vi "classes.vi"(0 "HGF_FGV_Factory":refnum<class "HGF_FGV_Factory.lvclass">, 1 "className":string, 5 "error in (no error)":errorcluster) -> (14 "dup HGF_FGV_Factory":refnum<class "HGF_FGV_Factory.lvclass">, 16 "Object":refnum<class>, 19 "error out":errorcluster)   [LabVIEW 2012, in "HGF_FGV.lvlib" / "HGF_FGV_Factory.lvclass"]
doc: "This dynamaic dispatch VI contains constant objects of all classes that can be produced by HGF_Factory.\nClass has to be defined by name. \n\nOptionally, you can also specifiy a Class Path String instead, but you have to make sure that all dependencies are available.\n\nChild classes have to override it to define additional classes."
uses:
  HGF_FGV_Factory.lvclass
  HGF_FGV_Append/HGF_FGV_Append.lvclass
  HGF_FGV_Clear/HGF_FGV_Clear.lvclass
  HGF_FGV_Delete/HGF_FGV_Delete.lvclass
  HGF_FGV_Index/HGF_FGV_Index.lvclass
  HGF_FGV_Insert/HGF_FGV_Insert.lvclass
  HGF_FGV_Replace/HGF_FGV_Replace.lvclass
  HGF_FGV_SelectByName/HGF_FGV_SelectByName.lvclass
  HGF_FGV_Selection/HGF_FGV_Selection.lvclass
  HGF_FGV_Size/HGF_FGV_Size.lvclass
  HGF_FGV_Subset/HGF_FGV_SubSet.lvclass
  HGF_FGV_VisitAll/HGF_FGV_VisitAll.lvclass
  HGF_FGV_VisitByName/HGF_FGV_VisitByName.lvclass
  HGF_FGV_VisitSelection/HGF_FGV_VisitSelection.lvclass
  HGF_FGV_VisitSubset/HGF_FGV_VisitSubSet.lvclass
  HGF_Factory/HGF_Factory.lvclass
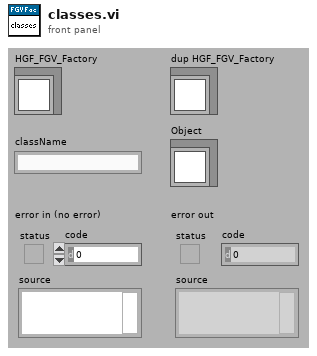
[diagram p1: front panel]
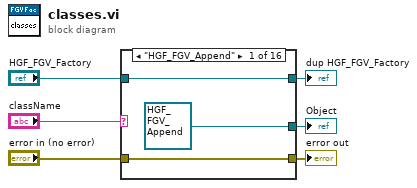
[diagram p0: block diagram]
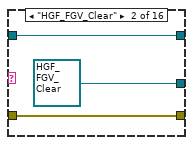
[diagram p2: hidden frame]
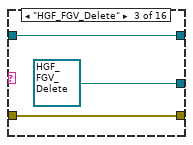
[diagram p3: hidden frame]
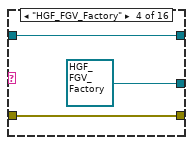
[diagram p4: hidden frame]
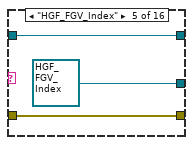
[diagram p5: hidden frame]
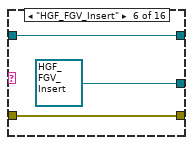
[diagram p6: hidden frame]
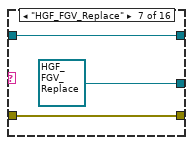
[diagram p7: hidden frame]
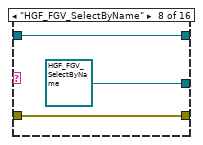
[diagram p8: hidden frame]
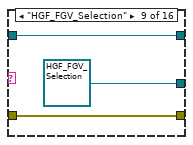
[diagram p9: hidden frame]
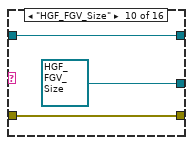
[diagram p10: hidden frame]
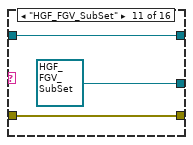
[diagram p11: hidden frame]
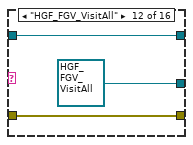
[diagram p12: hidden frame]
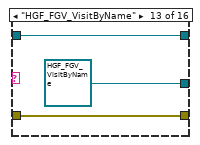
[diagram p13: hidden frame]
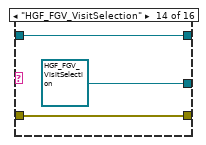
[diagram p14: hidden frame]
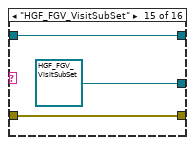
[diagram p15: hidden frame]
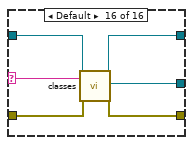
[diagram p16: hidden frame]
diagram:
  n1 = case shown="\"HGF_FGV_Append\"" "className" {
    selector: "className" -> [_ _ _ _ _ _ _ _ _ _ _ _ _ _ _ w54]
    tunnel: [refnum<class "HGF_FGV_Append.lvclass"> refnum ("HGF_FGV.lvlib:HGF_FGV_Append.lvclass") refnum<class "HGF_FGV_Clear.lvclass"> refnum ("HGF_FGV.lvlib:HGF_FGV_Clear.lvclass") refnum<class "HGF_FGV_Delete.lvclass"> refnum ("HGF_FGV.lvlib:HGF_FGV_Delete.lvclass") refnum<class "HGF_FGV_Factory.lvclass"> refnum ("HGF_FGV.lvlib:HGF_FGV_Factory.lvclass") refnum<class "HGF_FGV_Index.lvclass"> refnum ("HGF_FGV.lvlib:HGF_FGV_Index.lvclass") refnum<class "HGF_FGV_Insert.lvclass"> refnum ("HGF_FGV.lvlib:HGF_FGV_Insert.lvclass") refnum<class "HGF_FGV_Replace.lvclass"> refnum ("HGF_FGV.lvlib:HGF_FGV_Replace.lvclass") refnum<class "HGF_FGV_SelectByName.lvclass"> refnum ("HGF_FGV.lvlib:HGF_FGV_SelectByName.lvclass") refnum<class "HGF_FGV_Selection.lvclass"> refnum ("HGF_FGV.lvlib:HGF_FGV_Selection.lvclass") refnum<class "HGF_FGV_Size.lvclass"> refnum ("HGF_FGV.lvlib:HGF_FGV_Size.lvclass") refnum<class "HGF_FGV_SubSet.lvclass"> refnum ("HGF_FGV.lvlib:HGF_FGV_SubSet.lvclass") refnum<class "HGF_FGV_VisitAll.lvclass"> refnum ("HGF_FGV.lvlib:HGF_FGV_VisitAll.lvclass") refnum<class "HGF_FGV_VisitByName.lvclass"> refnum ("HGF_FGV.lvlib:HGF_FGV_VisitByName.lvclass") refnum<class "HGF_FGV_VisitSelection.lvclass"> refnum ("HGF_FGV.lvlib:HGF_FGV_VisitSelection.lvclass") refnum<class "HGF_FGV_VisitSubSet.lvclass"> refnum ("HGF_FGV.lvlib:HGF_FGV_VisitSubSet.lvclass") w55] -> w3
    tunnel: "error in (no error)" -> [w7 w10 w13 w17 w19 w22 w25 w28 w31 w34 w37 w40 w43 w46 w49 w57]
    tunnel: [w7 w10 w13 w17 w19 w22 w25 w28 w31 w34 w37 w40 w43 w46 w49 w56] -> w5
    tunnel: "HGF_FGV_Factory" -> [w8 w11 w14 w18 w20 w23 w26 w29 w32 w35 w38 w41 w44 w47 w50 w53]
    tunnel: [w8 w11 w14 w18 w20 w23 w26 w29 w32 w35 w38 w41 w44 w47 w50 w52] -> w1
    frame "HGF_FGV_Append" {
    }
    frame "HGF_FGV_Clear" {
    }
    frame "HGF_FGV_Delete" {
    }
    frame "HGF_FGV_Factory" {
    }
    frame "HGF_FGV_Index" {
    }
    frame "HGF_FGV_Insert" {
    }
    frame "HGF_FGV_Replace" {
    }
    frame "HGF_FGV_SelectByName" {
    }
    frame "HGF_FGV_Selection" {
    }
    frame "HGF_FGV_Size" {
    }
    frame "HGF_FGV_SubSet" {
    }
    frame "HGF_FGV_VisitAll" {
    }
    frame "HGF_FGV_VisitByName" {
    }
    frame "HGF_FGV_VisitSelection" {
    }
    frame "HGF_FGV_VisitSubSet" {
    }
    frame Default {
      n2 = call-parent "classes.vi"("HGF_Factory"=w53, "className"=w54, "error in (no error)"=w57) -> ("HGF_Factory dup"=w52:refnum<class "HGF_FGV_Factory.lvclass">, "Object"=w55:refnum<class>, "error out"=w56:errorcluster)  [unwired: 14 out]
    }
  }
  "error out" <- w5
  "dup HGF_FGV_Factory" <- w1
  "Object" <- w3
